vi "LabVIEWArduinoModbus.vi"() -> ()   [LabVIEW 2014]
uses:
  <vilib>/Modbus/master/Create Master Instance (Serial).vi
  <vilib>/Modbus/master/Modbus Master.lvclass
panel:
  in  "停止按钮":bool
  out "error out":errorcluster caption="错误输出"
  in  "coil value":bool caption="线圈值"
  in  "address":u16=13 caption="地址"
  in  "error in (no error)":errorcluster caption="错误输入（无错误）"
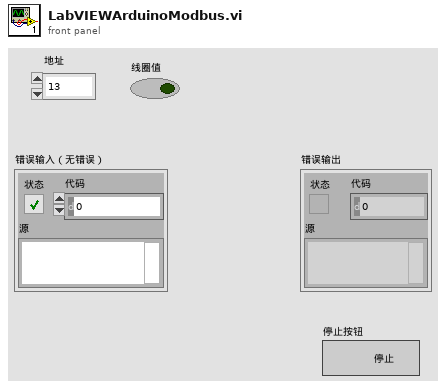
[diagram p1: front panel]
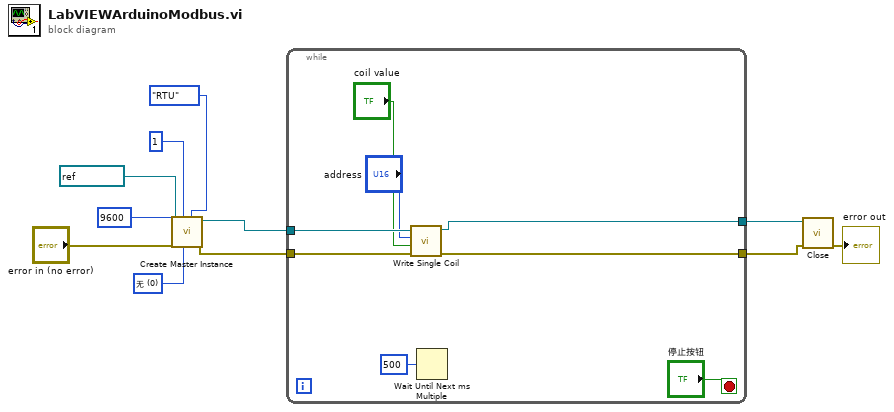
[diagram p0: block diagram]
diagram:
  w7 = u16 0 items=["无", "奇", "偶"] ("parity (Even)")
  n1 = call-poly <vilib>:"Create Master Instance.vi"("serial type"=enum16{"RTU", "ASCII"}."RTU", "parity (Even)"=w7, "unit ID"=u8 1, "error in (no error)"="error in (no error)", "baud rate (9600)"=u32 9600, "VISA resource name"=refnum<visa-resource-name> "COM3") -> ("error out"=w5:errorcluster, "serial master instance"=w6:refnum<class "Modbus Master.lvclass">)  [unwired: 4 in]
  n2 = while {
    tunnel: w6 -> [w19]
    tunnel: w5 -> [w16]
    tunnel: [w14] -> w3
    tunnel: [w13] -> w2
    stop <- "停止按钮" stop-if-true
    n3 = call-dynamic "Write Single Coil.vi"("error in (no error)"=w16, "coil value"="coil value", "address"="address", "Modbus master in"=w19) -> ("error out"=w14:errorcluster, "Modbus master out"=w13:refnum<class "Modbus Master.lvclass">)  [unwired: 6 in]
    n4 = Wait Until Next ms Multiple(millisecond multiple=u32 500 ("毫秒倍数")) -> ()  [unwired: 1 out]
  }
  n5 = call-dynamic "Close.vi"("error in (no error)"=w3, "Modbus master in"=w2) -> ("error out"=→"error out":errorcluster)  [unwired: 9 in]
